vi "数据编码整合输出.vi"(5 "table":string="N", 7 "数据标识":string="N", 8 "数据类型":string(combo)="-Rtd=", 9 "污染物编码":string, 10 "地表水/污染源":bool, 11 "数据值":string) -> (0 "编码输出":string)   [LabVIEW 2016, in "数据传输系统-02.lvlib"]
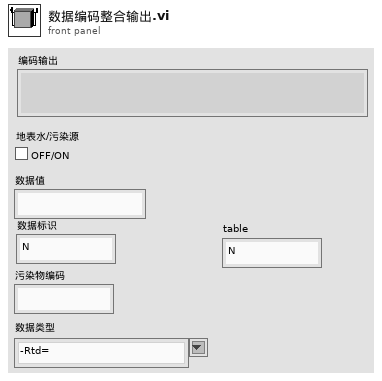
[diagram p1: front panel]
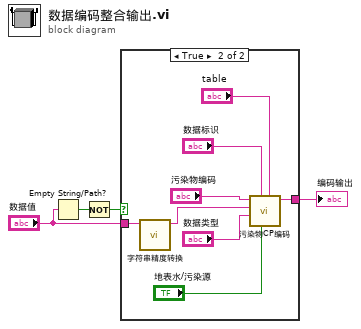
[diagram p0: block diagram]
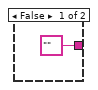
[diagram p2: hidden frame]
diagram:
  n1 = Empty String/Path?(string/path="数据值") -> (empty?=w2:bool)
  n2 = Not(x=w2) -> (.not. x?=w4:bool)
  n3 = case shown="True" w4 {
    tunnel: ["" ("编码输出") w13] -> w1
    tunnel: "数据值" -> [_ w10]
    frame False {
    }
    frame True {
      n4 = call "字符串精度转换.vi"("输入字符串"=w10) -> ("输出字符串"=w9:string)  [unwired: 9 in, 1 out]
      n5 = call "污染物CP编码.vi"("table"="table", "地表水/污染源"="地表水/污染源", "字符串"="数据标识", "数据类型"="数据类型", "污染物浓度"=w9, "污染物编码"="污染物编码") -> ("编码输出"=w13:string)  [unwired: 5 in]
    }
  }
  "编码输出" <- w1
